vi "getChannels.vi"(8 "error in (no error)":errorcluster, 11 "IDevice in":refnum<class "IDevice.lvclass">) -> (0 "error out":errorcluster, 2 "Channels out":refnum<class "IChannel.lvclass">[](array[class]), 3 "IDevice out":refnum<class "IDevice.lvclass">)   [LabVIEW 2022 SP3, in "openDAQ.lvlib" / "IBaseObject.lvlib" / "IPropertyObject.lvlib" / "IComponent.lvlib" / "IFolder.lvlib" / "IDevice.lvlib" / "IDevice.lvclass"]
uses:
  <instrlib>/openDAQ/Public/Classes/IDevice/IDevice.lvclass
  <instrlib>/openDAQ/Public/Classes/IDevice/IDevice.lvclass/IDevice.ctl
  <instrlib>/openDAQ/Public/Classes/daqCoreTypes/IList/IList.lvclass
  <instrlib>/openDAQ/Public/Classes/daqCoreTypes/IList/Polymorphic/getList/getChannelList.vi
  <instrlib>/openDAQ/Binaries/Windows/x86/copendaq32.dll
  <instrlib>/openDAQ/Public/Classes/IChannel/IChannel.lvclass
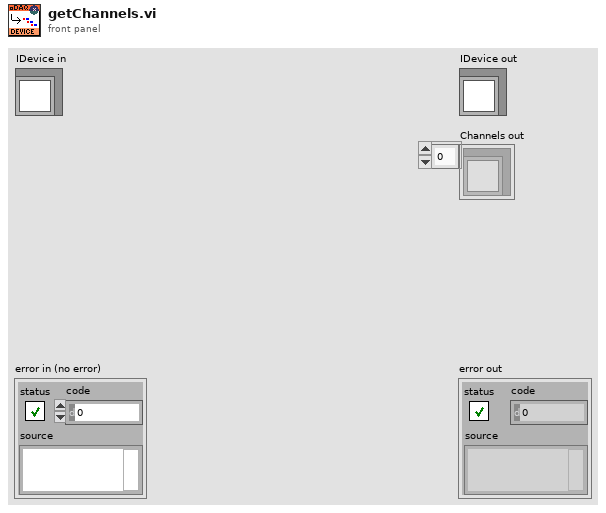
[diagram p1: front panel]
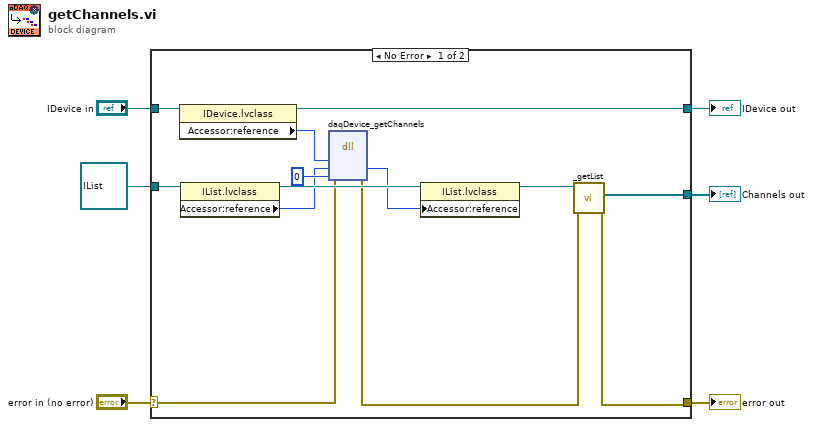
[diagram p0: block diagram]
diagram:
  n1 = case shown="No Error" "error in (no error)" {
    selector: "error in (no error)" -> [w11 w21]
    tunnel: [w7 w21] -> w5
    tunnel: [w16 w20] -> w3
    tunnel: "IDevice in" -> [w17 w20]
    tunnel: refnum<class "IList.lvclass"> refnum ("openDAQ.lvlib:daqCoreTypes.lvlib:IList.lvclass") -> [w14 _]
    tunnel: [w9 _] -> w1
    frame No Error {
      n2 = property class="IDevice.lvclass"(reference=w17) -> (reference out=w16:refnum<class "IDevice.lvclass">, "Accessor:reference"=w15:i64)  [unwired: 1 in, 1 out]
      n3 = property class="IList.lvclass"(reference=w14) -> (reference out=w18:refnum<class "IList.lvclass">, "Accessor:reference"=w13:i64)  [unwired: 1 in, 1 out]
      n4 = dll-call lib="C:/Program Files (x86)/National Instruments/LabVIEW 2022/instr.lib/openDAQ/Binaries/Windows/x86/copendaq*.*" fn="daqDevice_getChannels"(error in=w11, "instance"=w15, "channels"=w13, "searchFilter"=i64 0) -> (error out=w8:errorcluster, "channels"=w12:i64)  [unwired: 5 in, 1 out]
      n5 = property class="IList.lvclass"(reference=w18, "Accessor:reference"=w12) -> (reference out=w10:refnum<class "IList.lvclass">)  [unwired: 1 in, 1 out]
      n6 = call-poly <instrlib>:"_getList.vi"("error in (no error)"=w8, "IList in"=w10) -> ("error out"=w7:errorcluster, "devices out"=w9:refnum<class "IChannel.lvclass">[])  [unwired: 8 in]
    }
    frame Error {
    }
  }
  "error out" <- w5
  "IDevice out" <- w3
  "Channels out" <- w1
